vi "Мультиплексор(16 одноразрядных операндов).vi"(1 "c":T2, 2 "in":T1) -> (0 "r":bool)   [LabVIEW 2013]
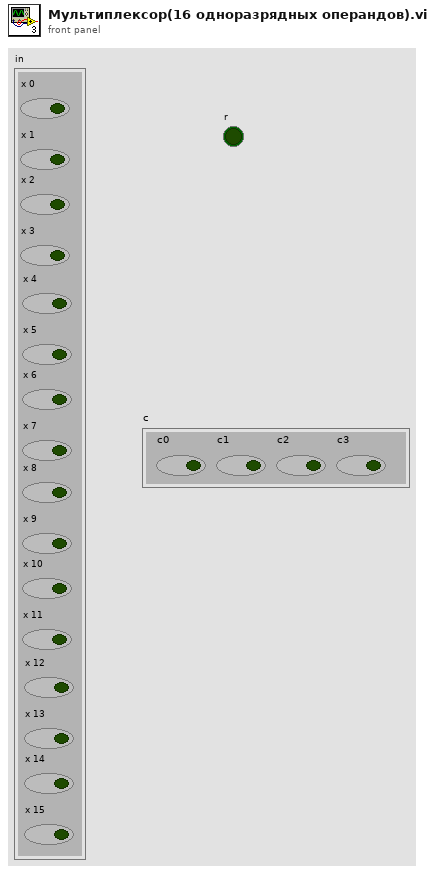
[diagram p1: front panel]
types:
  T1 = cluster{"x 0":bool, "x 1":bool, "x 2":bool, "x 3":bool, "x 4":bool, "x 5":bool, "x 6":bool, "x 7":bool, "x 8":bool, "x 9":bool, "x 10":bool, "x 11":bool, "x 12":bool, "x 13":bool, "x 14":bool, "x 15":bool}
  T2 = cluster{"c0":bool, "c1":bool, "c2":bool, "c3":bool}
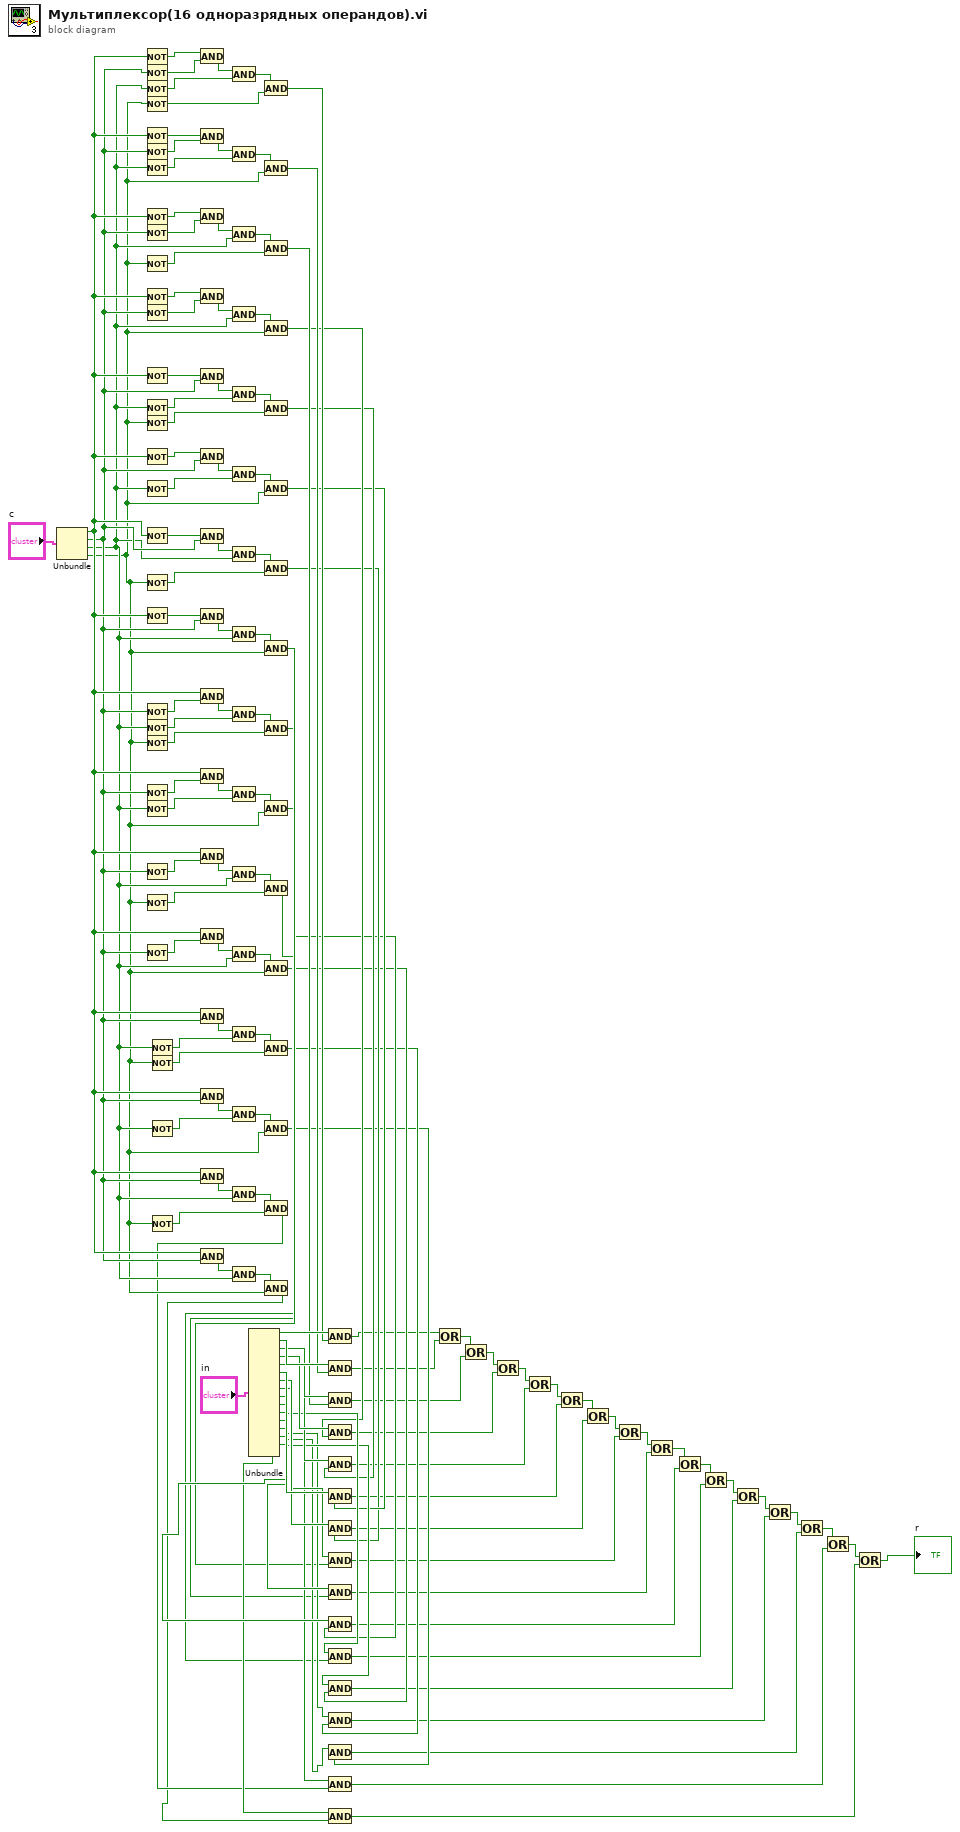
[diagram p0: block diagram]
diagram:
  n1 = Unbundle("c") -> ("c0"=w68:bool, "c1"=w67:bool, "c2"=w66:bool, "c3"=w65:bool)
  n2 = Not(x=w68) -> (.not. x?=w100:bool)
  n3 = Not(x=w67) -> (.not. x?=w99:bool)
  n4 = Not(x=w66) -> (.not. x?=w98:bool)
  n5 = Not(x=w65) -> (.not. x?=w97:bool)
  n6 = Not(x=w68) -> (.not. x?=w96:bool)
  n7 = Not(x=w67) -> (.not. x?=w95:bool)
  n8 = Not(x=w66) -> (.not. x?=w94:bool)
  n9 = Not(x=w68) -> (.not. x?=w93:bool)
  n10 = Not(x=w67) -> (.not. x?=w92:bool)
  n11 = Not(x=w65) -> (.not. x?=w91:bool)
  n12 = Not(x=w68) -> (.not. x?=w90:bool)
  n13 = Not(x=w67) -> (.not. x?=w89:bool)
  n14 = Not(x=w68) -> (.not. x?=w88:bool)
  n15 = Not(x=w66) -> (.not. x?=w87:bool)
  n16 = Not(x=w65) -> (.not. x?=w86:bool)
  n17 = Not(x=w68) -> (.not. x?=w85:bool)
  n18 = Not(x=w66) -> (.not. x?=w84:bool)
  n19 = Not(x=w68) -> (.not. x?=w83:bool)
  n20 = Not(x=w65) -> (.not. x?=w82:bool)
  n21 = Not(x=w68) -> (.not. x?=w81:bool)
  n22 = Not(x=w67) -> (.not. x?=w80:bool)
  n23 = Not(x=w66) -> (.not. x?=w79:bool)
  n24 = Not(x=w65) -> (.not. x?=w78:bool)
  n25 = Not(x=w67) -> (.not. x?=w77:bool)
  n26 = Not(x=w66) -> (.not. x?=w76:bool)
  n27 = Not(x=w67) -> (.not. x?=w75:bool)
  n28 = Not(x=w65) -> (.not. x?=w74:bool)
  n29 = Not(x=w67) -> (.not. x?=w73:bool)
  n30 = Not(x=w66) -> (.not. x?=w72:bool)
  n31 = Not(x=w65) -> (.not. x?=w71:bool)
  n32 = Not(x=w66) -> (.not. x?=w70:bool)
  n33 = Not(x=w65) -> (.not. x?=w69:bool)
  n34 = And(x=w100, y=w99) -> (x .and. y?=w132:bool)
  n35 = And(x=w96, y=w95) -> (x .and. y?=w130:bool)
  n36 = And(x=w93, y=w92) -> (x .and. y?=w128:bool)
  n37 = And(x=w90, y=w89) -> (x .and. y?=w126:bool)
  n38 = And(x=w88, y=w67) -> (x .and. y?=w124:bool)
  n39 = And(x=w85, y=w67) -> (x .and. y?=w122:bool)
  n40 = And(x=w83, y=w67) -> (x .and. y?=w120:bool)
  n41 = And(x=w81, y=w67) -> (x .and. y?=w118:bool)
  n42 = And(x=w68, y=w80) -> (x .and. y?=w116:bool)
  n43 = And(x=w68, y=w77) -> (x .and. y?=w114:bool)
  n44 = And(x=w68, y=w75) -> (x .and. y?=w112:bool)
  n45 = And(x=w68, y=w73) -> (x .and. y?=w110:bool)
  n46 = And(x=w68, y=w67) -> (x .and. y?=w108:bool)
  n47 = And(x=w68, y=w67) -> (x .and. y?=w106:bool)
  n48 = And(x=w68, y=w67) -> (x .and. y?=w104:bool)
  n49 = And(x=w68, y=w67) -> (x .and. y?=w102:bool)
  n50 = And(x=w132, y=w98) -> (x .and. y?=w131:bool)
  n51 = And(x=w130, y=w94) -> (x .and. y?=w129:bool)
  n52 = And(x=w128, y=w66) -> (x .and. y?=w127:bool)
  n53 = And(x=w126, y=w66) -> (x .and. y?=w125:bool)
  n54 = And(x=w124, y=w87) -> (x .and. y?=w123:bool)
  n55 = And(x=w122, y=w84) -> (x .and. y?=w121:bool)
  n56 = And(x=w120, y=w66) -> (x .and. y?=w119:bool)
  n57 = And(x=w118, y=w66) -> (x .and. y?=w117:bool)
  n58 = And(x=w116, y=w79) -> (x .and. y?=w115:bool)
  n59 = And(x=w114, y=w76) -> (x .and. y?=w113:bool)
  n60 = And(x=w112, y=w66) -> (x .and. y?=w111:bool)
  n61 = And(x=w110, y=w66) -> (x .and. y?=w109:bool)
  n62 = And(x=w108, y=w72) -> (x .and. y?=w107:bool)
  n63 = And(x=w106, y=w70) -> (x .and. y?=w105:bool)
  n64 = And(x=w104, y=w66) -> (x .and. y?=w103:bool)
  n65 = And(x=w102, y=w66) -> (x .and. y?=w101:bool)
  n66 = Unbundle("in") -> ("x 0"=w63:bool, "x 1"=w62:bool, "x 2"=w61:bool, "x 3"=w60:bool, "x 4"=w59:bool, "x 5"=w58:bool, "x 6"=w57:bool, "x 7"=w56:bool, "x 8"=w55:bool, "x 9"=w54:bool, "x 10"=w53:bool, "x 11"=w52:bool, "x 12"=w51:bool, "x 13"=w50:bool, "x 14"=w49:bool, "x 15"=w48:bool)
  n67 = And(x=w131, y=w97) -> (x .and. y?=w47:bool)
  n68 = And(x=w129, y=w65) -> (x .and. y?=w46:bool)
  n69 = And(x=w127, y=w91) -> (x .and. y?=w45:bool)
  n70 = And(x=w125, y=w65) -> (x .and. y?=w44:bool)
  n71 = And(x=w123, y=w86) -> (x .and. y?=w43:bool)
  n72 = And(x=w121, y=w65) -> (x .and. y?=w42:bool)
  n73 = And(x=w119, y=w82) -> (x .and. y?=w41:bool)
  n74 = And(x=w117, y=w65) -> (x .and. y?=w40:bool)
  n75 = And(x=w115, y=w78) -> (x .and. y?=w39:bool)
  n76 = And(x=w113, y=w65) -> (x .and. y?=w38:bool)
  n77 = And(x=w111, y=w74) -> (x .and. y?=w37:bool)
  n78 = And(x=w109, y=w65) -> (x .and. y?=w36:bool)
  n79 = And(x=w107, y=w71) -> (x .and. y?=w35:bool)
  n80 = And(x=w105, y=w65) -> (x .and. y?=w34:bool)
  n81 = And(x=w103, y=w69) -> (x .and. y?=w33:bool)
  n82 = And(x=w101, y=w65) -> (x .and. y?=w32:bool)
  n83 = And(x=w63, y=w47) -> (x .and. y?=w17:bool)
  n84 = And(x=w62, y=w46) -> (x .and. y?=w16:bool)
  n85 = And(x=w61, y=w45) -> (x .and. y?=w15:bool)
  n86 = And(x=w60, y=w44) -> (x .and. y?=w14:bool)
  n87 = And(x=w59, y=w43) -> (x .and. y?=w13:bool)
  n88 = And(x=w58, y=w42) -> (x .and. y?=w12:bool)
  n89 = And(x=w57, y=w41) -> (x .and. y?=w11:bool)
  n90 = And(x=w56, y=w40) -> (x .and. y?=w10:bool)
  n91 = And(x=w55, y=w39) -> (x .and. y?=w9:bool)
  n92 = And(x=w54, y=w38) -> (x .and. y?=w8:bool)
  n93 = And(x=w53, y=w37) -> (x .and. y?=w7:bool)
  n94 = And(x=w52, y=w36) -> (x .and. y?=w6:bool)
  n95 = And(x=w51, y=w35) -> (x .and. y?=w5:bool)
  n96 = And(x=w50, y=w34) -> (x .and. y?=w4:bool)
  n97 = And(x=w49, y=w33) -> (x .and. y?=w3:bool)
  n98 = And(x=w48, y=w32) -> (x .and. y?=w2:bool)
  n99 = Or(x=w17, y=w16) -> (x .or. y?=w31:bool)
  n100 = Or(x=w31, y=w15) -> (x .or. y?=w30:bool)
  n101 = Or(x=w30, y=w14) -> (x .or. y?=w29:bool)
  n102 = Or(x=w29, y=w13) -> (x .or. y?=w28:bool)
  n103 = Or(x=w28, y=w12) -> (x .or. y?=w27:bool)
  n104 = Or(x=w27, y=w11) -> (x .or. y?=w26:bool)
  n105 = Or(x=w26, y=w10) -> (x .or. y?=w25:bool)
  n106 = Or(x=w25, y=w9) -> (x .or. y?=w24:bool)
  n107 = Or(x=w24, y=w8) -> (x .or. y?=w23:bool)
  n108 = Or(x=w23, y=w7) -> (x .or. y?=w22:bool)
  n109 = Or(x=w22, y=w6) -> (x .or. y?=w21:bool)
  n110 = Or(x=w21, y=w5) -> (x .or. y?=w20:bool)
  n111 = Or(x=w20, y=w4) -> (x .or. y?=w19:bool)
  n112 = Or(x=w19, y=w3) -> (x .or. y?=w18:bool)
  n113 = Or(x=w18, y=w2) -> (x .or. y?=→"r":bool)
